vi "AnalyticsParamCluster.vi"(8 "error in (no error)":errorcluster, 9 "Number of columns":i32, 10 "MeasurementData":T2(array[cluster])) -> (0 "error out":errorcluster, 2 "Initialization Data":T1, 3 "x-y":i32)   [LabVIEW 2019, in "Zen Analytics.lvlib" / "Zen Analytics.lvclass"]
uses:
  Zen Analytics.lvclass
  <userlib>/_OpenG.lib/array/array.llb/Remove Duplicates from 1D Array (I32)__ogtk.vi
types:
  T1 = cluster{"Measurement-ID":i32[], "Measurement Names":string[], "NominalValues":dbl[], "LSL":dbl[], "USL":dbl[], "LCL":dbl[], "UCL":dbl[]}
  T2 = cluster{"Measurement ID":i32, "Measurement Name":string, "Nominal Values":dbl, "LSL":dbl, "USL":dbl, "LCL":dbl, "UCL":dbl}[]
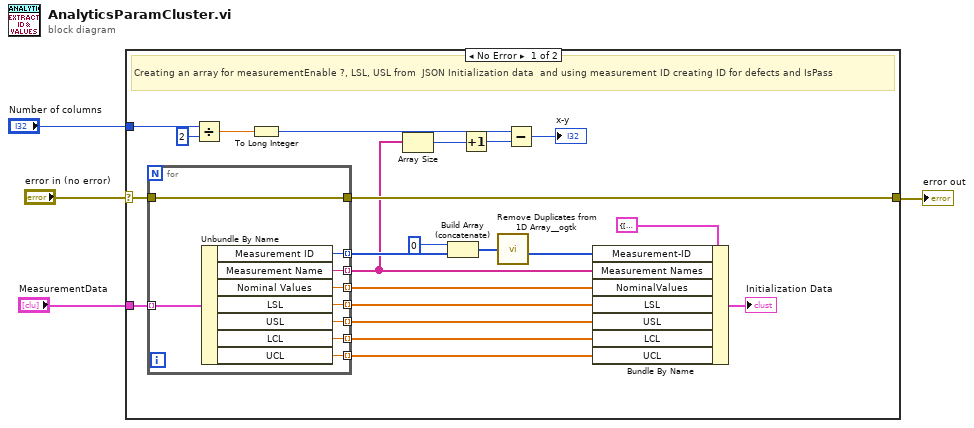
[diagram p0: block diagram]
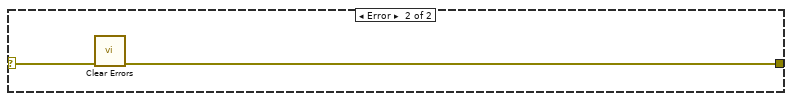
[diagram p2: hidden frame]
diagram:
  n1 = case shown="No Error" "error in (no error)" {
    selector: "error in (no error)" -> [w26 w37]
    tunnel: [w6 w36] -> w1
    tunnel: "MeasurementData" -> [w25 _]
    tunnel: "Number of columns" -> [w17 _]
    frame No Error {
      # "Creating an array for measurementEnable ?, LSL, USL from  JSON Initialization data  and using measurement ID creating ID for defects and IsPass"
      n2 = for {
        tunnel: w25 -> [w35] mode=indexing
        tunnel: [w34] -> w15 mode=indexing
        tunnel: [w33] -> w5 mode=indexing
        tunnel: [w32] -> w6
        tunnel: w26 -> [w32]
        tunnel: [w31] -> w22 mode=indexing
        tunnel: [w30] -> w21 mode=indexing
        tunnel: [w29] -> w20 mode=indexing
        tunnel: [w28] -> w19 mode=indexing
        tunnel: [w27] -> w10 mode=indexing
        n3 = Unbundle By Name(w35) -> ("Measurement ID"=w34:i32, "Measurement Name"=w33:string, "Nominal Values"=w31:dbl, "LSL"=w30:dbl, "USL"=w29:dbl, "LCL"=w28:dbl, "UCL"=w27:dbl)
      }
      n4 = Divide(x=w17, y=2) -> (x/y=w9:dbl)
      n5 = To Long Integer(number=w9) -> (32bit integer=w8:i32)
      n6 = Array Size(array=w5) -> (size(s)=w11:i32)
      n7 = Build Array (concatenate)(0 ("index"), w15) -> (w14:i32[])
      n8 = Increment(x=w11) -> (x+1=w12:i32)
      n9 = call-poly <userlib>:"Remove Duplicates from 1D Array__ogtk.vi"("Input Array"=w14) -> ("Output Array"=w13:i32[])  [unwired: 1 out]
      n10 = Subtract(x=w8, y=w12) -> (x-y=→"x-y":i32)
      n11 = Bundle By Name(cluster=T1 {"Measurement-ID"=[], "Measurement Names"=[], "NominalValues"=[], "LSL"=[], "USL"=[], "LCL"=[], "UCL"=[]} ("input cluster"), "Measurement-ID"=w13, "Measurement Names"=w5, "NominalValues"=w22, "LSL"=w21, "USL"=w20, "LCL"=w19, "UCL"=w10) -> (→"Initialization Data":T1)
    }
    frame Error {
      n12 = call <vilib>:"Clear Errors.vi"("error in (no error)"=w37) -> ("error out"=w36:errorcluster)  [unwired: 5 in, 1 out]
    }
  }
  "error out" <- w1
